vi "Clip AO Waveforms.vi"(8 "error in (no error)":errorcluster, 10 "AO []":waveform(dbl)[](array[waveform]), 11 "Instrument.DAQ in":refnum<class "Instrument.DAQ.lvclass">) -> (0 "error out":errorcluster, 2 "Clipped AO []":waveform(dbl)[](array[waveform]), 3 "Instrument.DAQ out":refnum<class "Instrument.DAQ.lvclass">)   [LabVIEW 2019, in "Instrument.Lockin.lvlib" / "Instrument.DAQ.lvclass"]
uses:
  Instrument.DAQ.lvclass
  Instrument.DAQ.lvclass/Instrument.DAQ.ctl
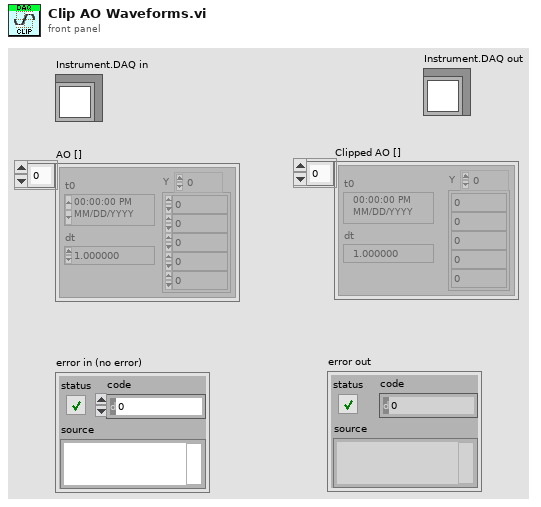
[diagram p1: front panel]
types:
  T1 = typedef "Instrument.Lockin.lvlib/Instrument.DAQ.lvclass/DAQ.Config.AO--Cluster--Array.ctl" = cluster{"Channels":tag, "Range":T2, "terminal configuration":T3, "Type":T4}[]
  T2 = typedef "Instrument.Lockin.lvlib/Instrument.DAQ.lvclass/DAQ.Config.AO.Range--enum.ctl" = enum16{"±0.1", "±1.0", "±10.0", ""}
  T3 = typedef "Instrument.Lockin.lvlib/Instrument.DAQ.lvclass/DAQ.TerminalConfiguration--ring.ctl" = i32
  T4 = typedef "Instrument.Lockin.lvlib/Instrument.DAQ.lvclass/DAQ.Type--enum.ctl" = enum16{"None", "USB-4431", "PXI-446x"}
  T5 = cluster{"Channels":tag, "Range":T2, "terminal configuration":T3, "Type":T4}
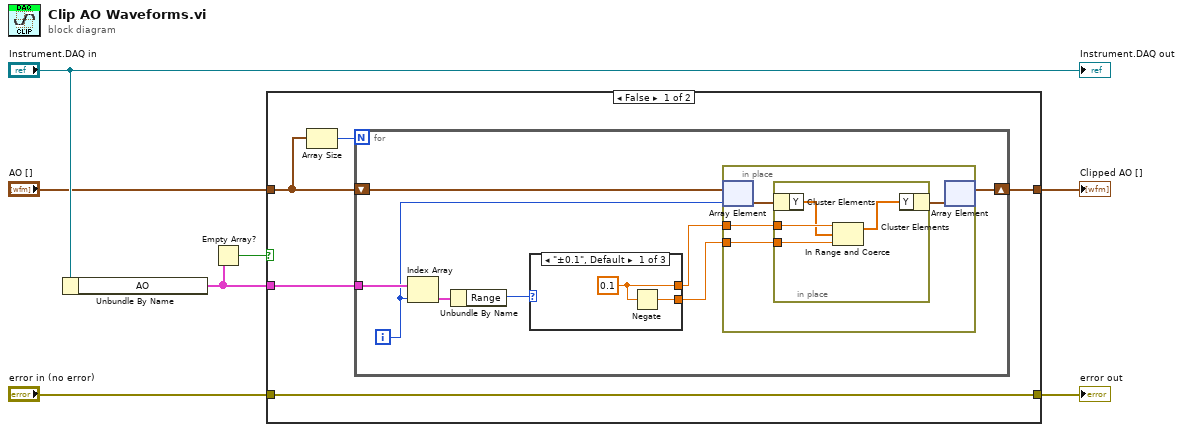
[diagram p0: block diagram]
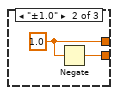
[diagram p2: hidden frame]
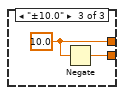
[diagram p3: hidden frame]
diagram:
  n1 = Unbundle By Name("Instrument.DAQ in") -> ("AO"=w1:T1)
  n2 = Empty Array?(array=w1) -> (empty?=w6:bool)
  n3 = case shown="False" w6 {
    tunnel: [w12 w36] -> w7
    tunnel: w1 -> [w8 _]
    tunnel: "error in (no error)" -> [w11 w35]
    tunnel: [w11 w35] -> w3
    tunnel: "AO []" -> [w9 w36]
    frame False {
      n4 = Array Size(array=w9) -> (size(s)=w10:i32)
      n5 = for {
        N: w10 -> [_]
        shift-right: [w19] -> w12
        shift-left: w9 -> [w20]
        tunnel: w8 -> [w16]
        i -> [w14]
        n6 = Index Array(array=w16, index=w14) -> (element=w15:T5)
        n7 = Unbundle By Name(w15) -> ("Range"=w18:T2)
        n8 = case shown="\"±0.1\", Default" w18 {
          tunnel: [w22 w24 w26] -> w17
          tunnel: [w21 w23 w25] -> w13
          frame "±0.1", Default {
            w22 = 0.1
            n9 = Negate(x=w22) -> (-x=w21:dbl)
          }
          frame "±1.0" {
            w24 = 1.0
            n10 = Negate(x=w24) -> (-x=w23:dbl)
          }
          frame "±10.0" {
            w26 = 10.0
            n11 = Negate(x=w26) -> (-x=w25:dbl)
          }
        }
        n12 = in-place {
          in-place-border: w17 -> [w30]
          in-place-border: w13 -> [w29]
          n13 = in-place-array #1(w20, w14) -> (w28:waveform(dbl))
          n14 = in-place {
            in-place-border: w30 -> [w34]
            in-place-border: w29 -> [w33]
            n15 = in-place-cluster #2(w28) -> ("Y"=w32:dbl[])
            n16 = In Range and Coerce(upper limit=w34, x=w32, lower limit=w33) -> (coerced(x)=w31:dbl[])  [unwired: 1 out]
            n17 = in-place-cluster #2("Y"=w31) -> (w27:waveform(dbl))
          }
          n18 = in-place-array #1(w27) -> (w19:waveform(dbl)[])  [unwired: 1 out]
        }
      }
    }
    frame True {
      # "If AO Config = empty, do nothing"
    }
  }
  "Clipped AO []" <- w7
  "error out" <- w3
  "Instrument.DAQ out" <- "Instrument.DAQ in"
